vi "MCL Read Value.vi"(8 "error in (no error)":errorcluster, 11 "MCL Ref (generic)":refnum<vi>) -> (0 "error out":errorcluster, 2 "Value":i32[](array[numeric]), 3 "MCL Ref (generic)":refnum<vi>)   [LabVIEW 2020, in "BetterDragAndDrop.lvlib" / "BetterMultiListboxHandle.lvclass"]
uses:
  BetterMultiListboxHandle.lvclass
  <vilib>/Utility/error.llb/Error Cluster From Error Code.vi
  <vilib>/ErrorRing/Error Ring.xnode
  BetterMultiListboxHandle.lvclass/BetterMultiListboxHandle.ctl
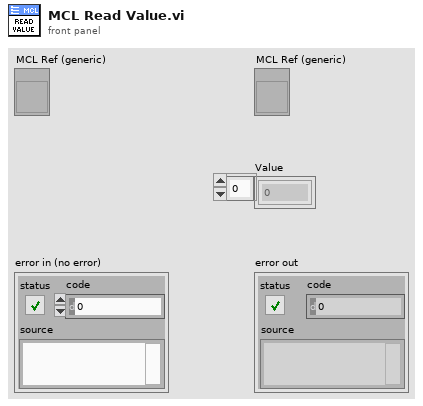
[diagram p1: front panel]
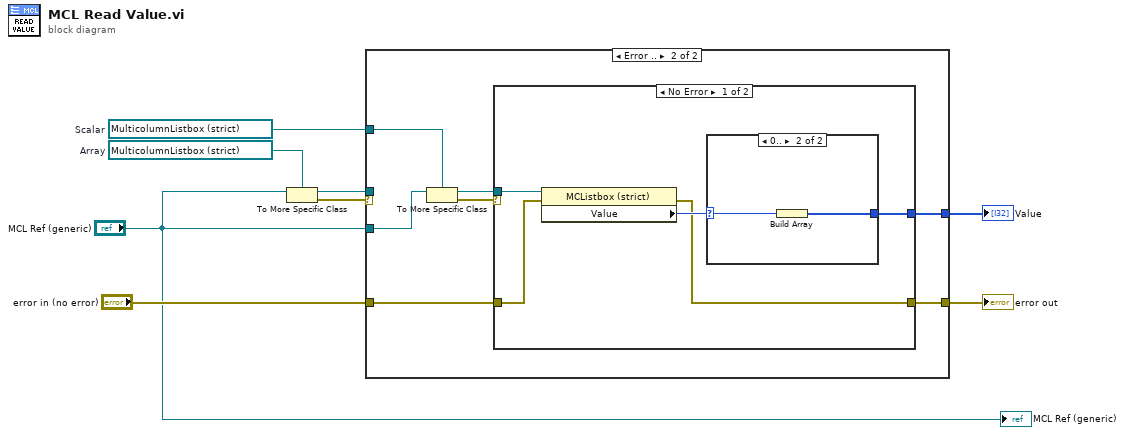
[diagram p0: block diagram]
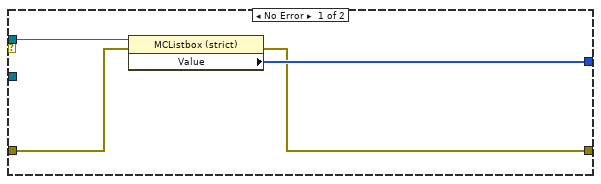
[diagram p2: hidden frame]
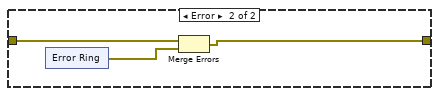
[diagram p4: hidden frame]
diagram:
  w8 = refnum<vi> refnum  # Array
  w5 = refnum<vi> refnum  # Scalar
  n1 = To More Specific Class(target class=w8, reference="MCL Ref (generic)") -> (specific class reference=w6:refnum<vi>, error out=w7:errorcluster)  [unwired: 1 in]
  n2 = case shown="Error .." w7 {
    tunnel: w6 -> [w12 _]
    tunnel: "MCL Ref (generic)" -> [_ w19]
    tunnel: w5 -> [_ w18]
    tunnel: "error in (no error)" -> [w10 w15]
    tunnel: [w9 w14] -> w3
    tunnel: [w11 w13] -> w2
    frame No Error {
      n3 = property class="MCListbox (strict)"(reference=w12, error in=w10) -> (error out=w9:errorcluster, "Value"=w11:i32[])  [unwired: 1 out]
    }
    frame Error {
      n4 = To More Specific Class(target class=w18, reference=w19) -> (specific class reference=w16:refnum<vi>, error out=w17:errorcluster)  [unwired: 1 in]
      n5 = case shown="No Error" w17 {
        tunnel: w16 -> [w24 _]
        tunnel: w15 -> [w21 w28]
        tunnel: [w20 w27] -> w14
        tunnel: [w22 _] -> w13
        frame No Error {
          n6 = property class="MCListbox (strict)"(reference=w24, error in=w21) -> (error out=w20:errorcluster, "Value"=w23:i32)  [unwired: 1 out]
          n7 = case shown="0.." w23 {
            selector: w23 -> [_ w26]
            tunnel: [_ w25] -> w22
            frame Default {
            }
            frame 0.. {
              n8 = Build Array(w26) -> (w25:i32[])
            }
          }
        }
        frame Error {
          n9 = xnode "Error Ring"() -> ("error out"=w29:errorcluster)
          n10 = Merge Errors(w28, w29) -> (w27:errorcluster)
        }
      }
    }
  }
  "error out" <- w3
  "Value" <- w2
  "MCL Ref (generic)" <- "MCL Ref (generic)"
